vi "Configure Pulse Waveform.vi"(5 "Trailing Edge Time (5.0E-8)":dbl=5e-08 format="%#.6g", 6 "Delay (0 s)":dbl, 7 "Leading Edge Time (5.0E-8)":dbl=5e-08 format="%#.6g", 8 "error in (no error)":errorcluster, 9 "Duty Cycle (50%)":dbl=50.0, 10 "Channel (0: Channel 1)":u16(ring) items=["Channel 1", "Channel 2"], 11 "VISA resource name":refnum<visa-resource-name>) -> (0 "error out":errorcluster, 3 "VISA resource name out":refnum<visa-resource-name>)   [LabVIEW 2018, in "AWG.lvlib" / "Tektronix AFG 3000 Series.lvlib"]
doc: "Configures parameters for pulse waveforms which include channel, leading edge time, trailing edge time, duty cycle, and delay."
uses:
  Tektronix AFG 3000 Series.lvlib
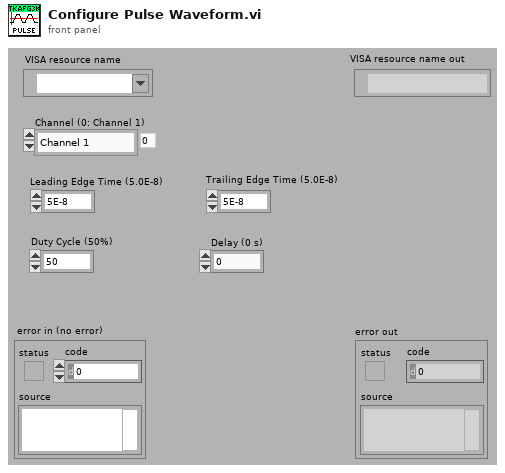
[diagram p1: front panel]
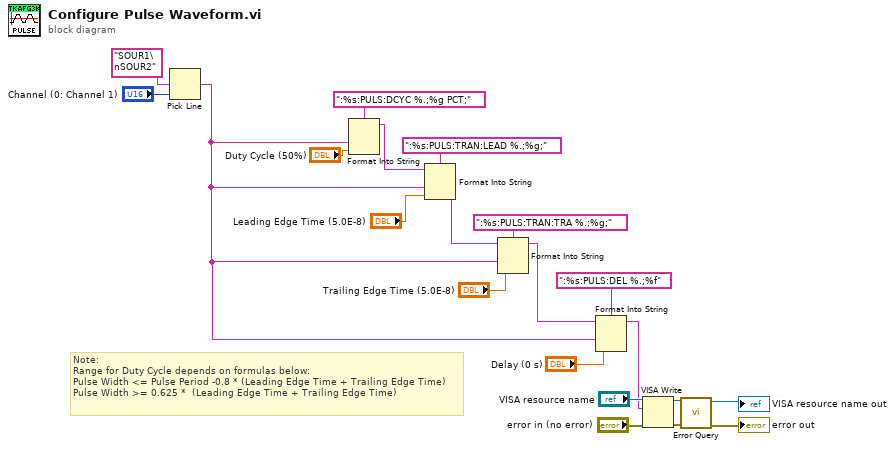
[diagram p0: block diagram]
diagram:
  # "Note:\nRange for Duty Cycle depends on formulas below:\nPulse Width <= Pulse Period -0.8 * (Leading Edge Time + Trailing Edge Time)\nPulse Width >= 0.625 *  (Leading Edge Time + Trailing Edge Time)"
  n1 = Pick Line(multi-line string="SOUR1\nSOUR2" ("string (\"\")"), line index="Channel (0: Channel 1)") -> (output string=w2:string)  [unwired: 1 in]
  n2 = Format Into String(format string=":%s:PULS:DCYC %.;%g PCT;", w2, "Duty Cycle (50%)") -> (resulting string=w14:string)  [unwired: 2 in, 1 out]
  n3 = Format Into String(format string=":%s:PULS:TRAN:LEAD %.;%g;", initial string=w14, w2, "Leading Edge Time (5.0E-8)") -> (resulting string=w13:string)  [unwired: 1 in, 1 out]
  n4 = Format Into String(format string=":%s:PULS:TRAN:TRA %.;%g;", initial string=w13, w2, "Trailing Edge Time (5.0E-8)") -> (resulting string=w4:string)  [unwired: 1 in, 1 out]
  n5 = Format Into String(format string=":%s:PULS:DEL %.;%f" ("string"), initial string=w4, w2, "Delay (0 s)") -> (resulting string=w1:string)  [unwired: 1 in, 1 out]
  n6 = VISA Write(VISA resource name="VISA resource name", write buffer=w1, error in (no error)="error in (no error)") -> (VISA resource name out=w19:refnum<visa-resource-name>, error out=w18:errorcluster)  [unwired: 1 out]
  n7 = call "Error Query.vi"("error in (no error)"=w18, "VISA resource name"=w19) -> ("error out"=→"error out":errorcluster, "VISA resource name out"=→"VISA resource name out":refnum<visa-resource-name>)  [unwired: 6 in, 2 out]
